vi "gxml_Generator.vi"(5 "Version String":string, 7 "Version Tag Name":string, 8 "error in":errorcluster, 10 "Variant":variant) -> (0 "error out":errorcluster, 2 "XML String Out":string)   [LabVIEW 2011, in "Third Party VIs.lvlib" / "GXML.lvlib"]
doc: "Using a custom XML schema, this VI converts LabVIEW data into an XML string. Data elements within any compound structure (such as multidimensional arrays, sub-clusters, or arrays of clusters) are represented with an appropriate hierarchy. The name of each LabVIEW control directly maps to the name of each XML element.\n\nEach control name must begin with a letter and adhere to XML specifications. No two controls of the same hierarchy may have the same name. Supported datatypes include integer, floating, complex, enum, boolean, string, path, and timestamp."
uses:
  GXML.lvlib
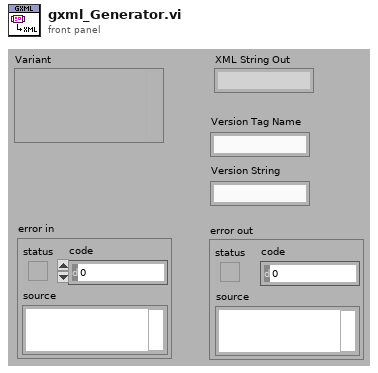
[diagram p1: front panel]
types:
  T1 = cluster{"In Empty Array?":bool, "Whitespace In":string}
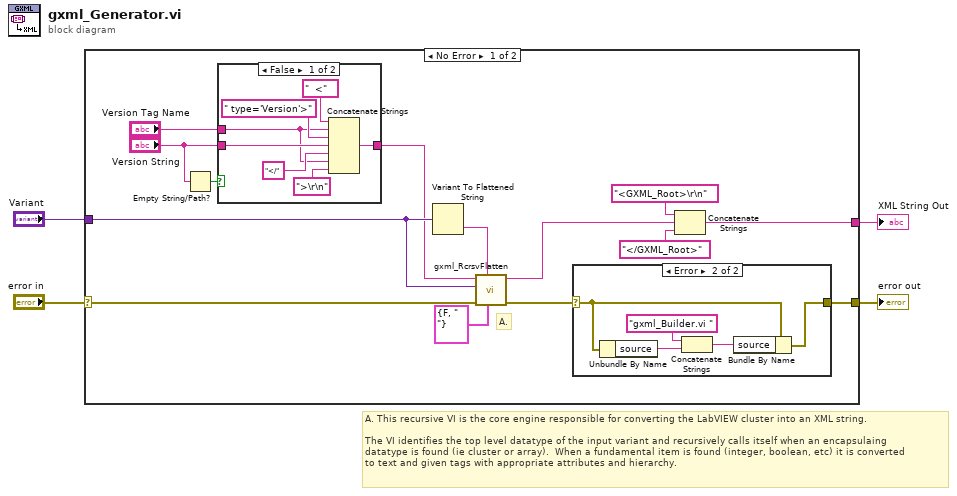
[diagram p0: block diagram]
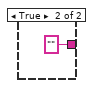
[diagram p2: hidden frame]
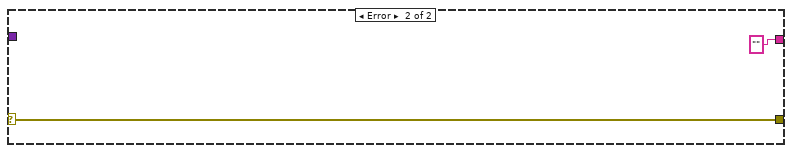
[diagram p4: hidden frame]
diagram:
  # "A. This recursive VI is the core engine responsible for converting the LabVIEW cluster into an XML string.  \n\nThe VI identifies the top level datatype of the input variant and recursively calls itself when an encapsulaing \ndatatype is found (ie cluster or array).  When a fundamental item is found (integer, boolean, etc) it is converted\nto text and given tags with appropriate attributes and hierarchy."
  n1 = case shown="No Error" "error in" {
    selector: "error in" -> [w15 w34]
    tunnel: [w12 "" ("XML String Out")] -> w4
    tunnel: "Variant" -> [w18 _]
    tunnel: [w16 w34] -> w2
    frame No Error {
      # "A."
      n2 = Empty String/Path?(string/path="Version String") -> (empty?=w9:bool)
      n3 = case shown="False" w9 {
        tunnel: "Version String" -> [w23 _]
        tunnel: "Version Tag Name" -> [w21 _]
        tunnel: [w19 ""] -> w8
        frame False {
          n4 = Concatenate Strings("  <" ("string"), w21, " type='Version'>" ("string"), w23, "</" ("string"), w21, ">\r\n" ("string")) -> (w19:string)
        }
        frame True {
        }
      }
      n5 = Variant To Flattened String(Variant=w18) -> (data string=w14:string)  [unwired: 1 out]
      n6 = call "gxml_RcrsvFlatten.vi"("HierarchyInfo"=T1 {"In Empty Array?"=FALSE, "Whitespace In"="  "}, "FlattenedData"=w14, "error in"=w15, "Variant"=w18, "XML String In"=w8) -> ("error out"=w17:errorcluster, "XML String Out"=w13:string)  [unwired: 4 in, 1 out]
      n7 = case shown="Error" w17 {
        selector: w17 -> [w27 w29]
        tunnel: [w27 w28] -> w16
        frame No Error {
        }
        frame Error {
          n8 = Unbundle By Name(w29) -> ("source"=w32:string)
          n9 = Concatenate Strings("gxml_Builder.vi ", w32) -> (w30:string)
          n10 = Bundle By Name(cluster=w29, "source"=w30) -> (w28:errorcluster)
        }
      }
      n11 = Concatenate Strings("<GXML_Root>\r\n" ("string"), w13, "</GXML_Root>" ("string")) -> (w12:string)
    }
    frame Error {
    }
  }
  "XML String Out" <- w4
  "error out" <- w2
